vi "QueryWavelength.vi"(8 "error in (no error)":errorcluster, 11 "DongWoo in":refnum<class "DongWoo.lvclass">) -> (0 "error out":errorcluster, 3 "DongWoo out":refnum<class "DongWoo.lvclass">)   [LabVIEW 2023, in "DongWoo_Spectrometer.lvlib" / "DongWoo.lvclass"]
uses:
  DongWoo.lvclass
  DongWoo.lvclass/DongWoo.ctl
  Interfaces/AbstractInstrumentClasses/Spectrometers_LV/SpectrometerComm Messages/WavelengthSet Msg/WavelengthSet Msg.lvclass
  <vilib>/ActorFramework/Actor/Actor.lvclass
  C:/Program Files/National Instruments/LabVIEW 2023/vi.lib/ActorFramework/Actor/Actor.lvclass
  C:/Users/DELL/Documents/LVDAQ/ConcreteClasses/ConcreteInstrumentClasses/SpectrometerClasses/DongWoo_LV/DongWoo/DongWoo.lvclass
  C:/Users/DELL/Documents/LVDAQ/Interfaces/InitDeinitInterface/InitDeinit/InitDeinit.lvclass
  C:/Users/DELL/Documents/LVDAQ/Interfaces/AbstractInstrumentClasses/Spectrometers_LV/SpectrometerInterface/Spectrometer.lvclass
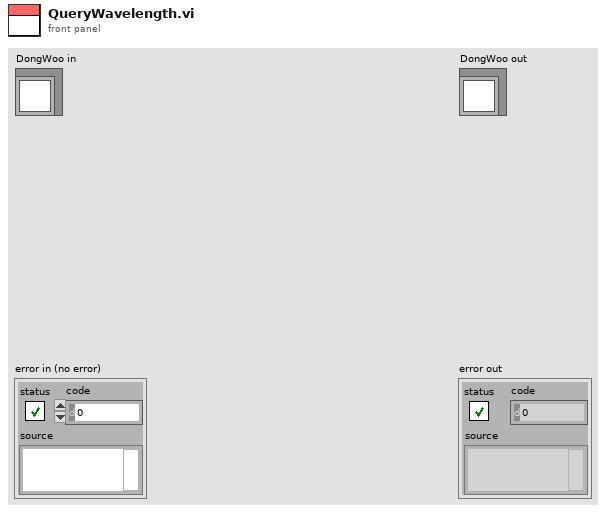
[diagram p1: front panel]
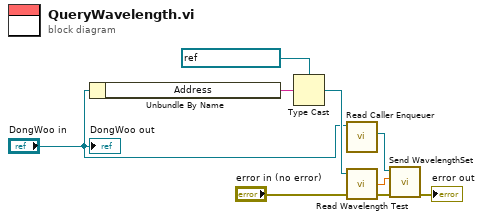
[diagram p0: block diagram]
diagram:
  n1 = Unbundle By Name("DongWoo in") -> ("Address"=w9:string)
  n2 = Type Cast(type=refnum<visa-resource-name> "ASRL1::INSTR" ("Resource Name"), x=w9) -> (*(type *) &x=w7:refnum<visa-resource-name>)
  n3 = call <vilib>:"Read Caller Enqueuer.vi"("Actor"="DongWoo in") -> ("Caller Enqueuer"=w4:refnum<class "Message Enqueuer.lvclass">)  [unwired: 10 in]
  n4 = call "Read Wavelength Test.vi"("Error In (no error)"="error in (no error)", "Resource Name"=w7) -> ("Error Out"=w2:errorcluster, "Wavelength"=w1:dbl)  [unwired: 1 in, 1 out]
  n5 = call "Send WavelengthSet.vi"("error in (no error)"=w2, "Wavelength"=w1, "Message Enqueuer"=w4) -> ("error out"=→"error out":errorcluster)  [unwired: 7 in, 1 out]
  "DongWoo out" <- "DongWoo in"
